vi "libssh2_knownhost_get.vi"(8 "error in (no error)":errorcluster, 10 "previous known host":T1, 11 "known hosts":T2) -> (0 "error out":errorcluster, 2 "next known host":T1, 3 "return value":i32)   [LabVIEW 2013, in "libssh2.lvlib"]
doc: "Gets a known host from the collection of known hosts."
uses:
  libssh2.lvlib
  Known Hosts Refnum.ctl
  Known Host Refnum.ctl
  Global Settings.vi
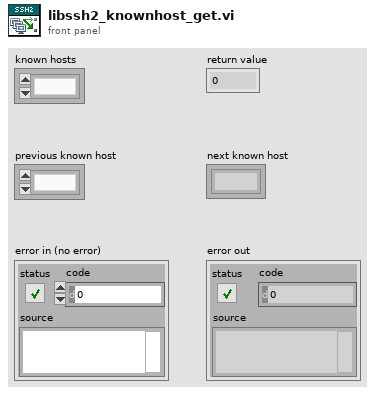
[diagram p1: front panel]
types:
  T1 = typedef "libssh2.lvlib/Known Host Refnum.ctl" = refnum<k1>
  T2 = typedef "libssh2.lvlib/Known Hosts Refnum.ctl" = refnum<k1>
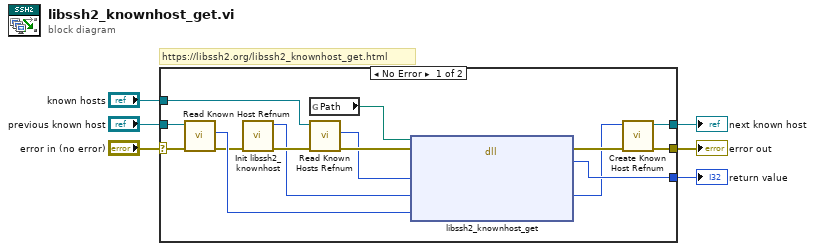
[diagram p0: block diagram]
diagram:
  # "https://libssh2.org/libssh2_knownhost_get.html"
  n1 = case shown="No Error" "error in (no error)" {
    selector: "error in (no error)" -> [w8 w22]
    tunnel: [w21 _] -> w6
    tunnel: [w19 w22] -> w5
    tunnel: "known hosts" -> [w17 _]
    tunnel: "previous known host" -> [w15 _]
    tunnel: [w13 _] -> w2
    frame No Error {
      n2 = call "Read Known Host Refnum.vi"("error in (no error)"=w8, "known host"=w15) -> ("error out"=w11:errorcluster, "libssh2_knownhost*"=w14:u64)  [unwired: 8 in]
      n3 = call "Init libssh2_knownhost.vi"("error in (no error)"=w11) -> ("error out"=w10:errorcluster, "libssh2_knownhost*"=w9:u64)  [unwired: 9 in]
      n4 = global read "Global Settings.vi" "Path"() -> (w7:path)
      n5 = call "Read Known Hosts Refnum.vi"("error in (no error)"=w10, "known hosts"=w17) -> ("error out"=w18:errorcluster, "LIBSSH2_KNOWNHOSTS*"=w16:u64)  [unwired: 8 in]
      n6 = dll-call lib="C:/Users/pasca/source/repos/libssh2-labview/libssh2/libssh2**.*" fn="libssh2_knownhost_get"(path in=w7, error in=w18, "hosts"=w16, "store"=w9, "prev"=w14) -> (error out=w20:errorcluster, "return value"=w21:i32, "store"=w12:u64)  [unwired: 3 in, 1 out]
      n7 = call "Create Known Host Refnum.vi"("error in (no error)"=w20, "libssh2_knownhost*"=w12) -> ("error out"=w19:errorcluster, "known host"=w13:T1)  [unwired: 8 in]
    }
    frame Error {
    }
  }
  "return value" <- w6
  "error out" <- w5
  "next known host" <- w2
